vi "Cluster Node_Has Unwired Elements.vi"(11 "Display Items":T1[](array[typedef])) -> (2 "Has unwired properties?":bool, 3 "Unwired Indicies":i32[](array[numeric]))   [LabVIEW 2023]
uses:
  Cluster Element Description.ctl
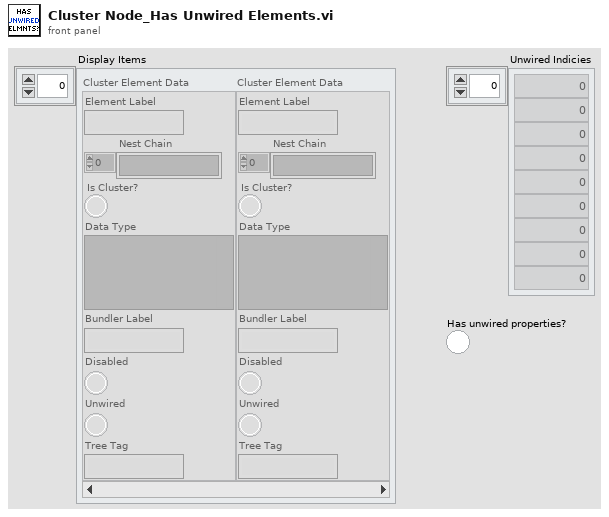
[diagram p1: front panel]
types:
  T1 = typedef "Cluster Element Description.ctl" = cluster{"Element Label":string, "Nest Chain":string[], "Is Cluster?":bool, "Data Type":variant, "Bundler Label":string, "Disabled":bool, "Unwired":bool, "Tree Tag":string}
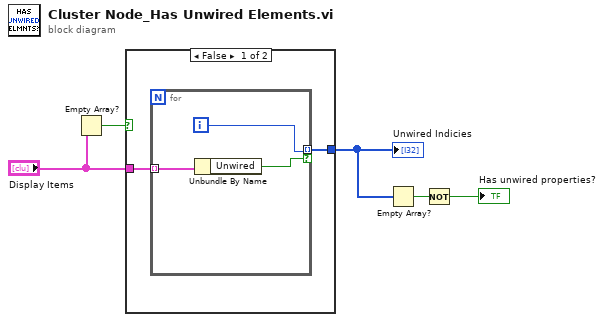
[diagram p0: block diagram]
diagram:
  n1 = Empty Array?(array="Display Items") -> (empty?=w2:bool)
  n2 = case shown="False" w2 {
    tunnel: "Display Items" -> [w7 _]
    tunnel: [w6 _] -> w4
    frame False {
      n3 = for {
        tunnel: w7 -> [w10] mode=indexing
        tunnel: [w8] -> w6 mode=indexing if=w9
        i -> [w8]
        n4 = Unbundle By Name(w10) -> ("Unwired"=w9:bool)
      }
    }
    frame True {
    }
  }
  "Unwired Indicies" <- w4
  n5 = Empty Array?(array=w4) -> (empty?=w3:bool)
  n6 = Not(x=w3) -> (.not. x?=→"Has unwired properties?":bool)
